vi "Pause.vi"(8 "error in (no error)":errorcluster, 11 "TDCManager":T1) -> (0 "error out":errorcluster, 3 "TDCManager":T1)   [LabVIEW 2016, in "HPTDC Driver Library.lvlib"]
uses:
  HPTDC Driver Library.lvlib
  Typedefs/TDCManager.ctl
  C:/Users/CRT Controller/CRTC Labview Application/Source/HPTDC Driver Library Folder/Library files/hptdc_net4_3.7.0_x64.dll
  hptdc_net4_3.7.0_x64.dll
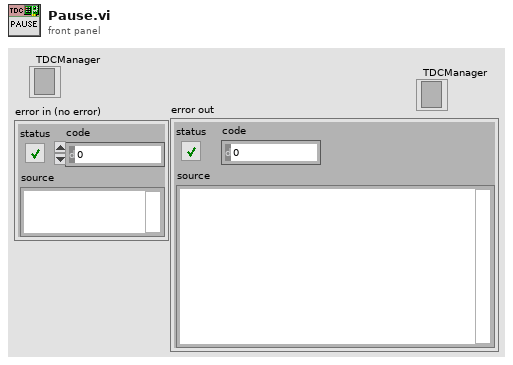
[diagram p1: front panel]
types:
  T1 = typedef "HPTDC Driver Library.lvlib/TDCManager.ctl" = refnum<k24>
  T2 = typedef "Semaphore RefNum" = refnum<k1>
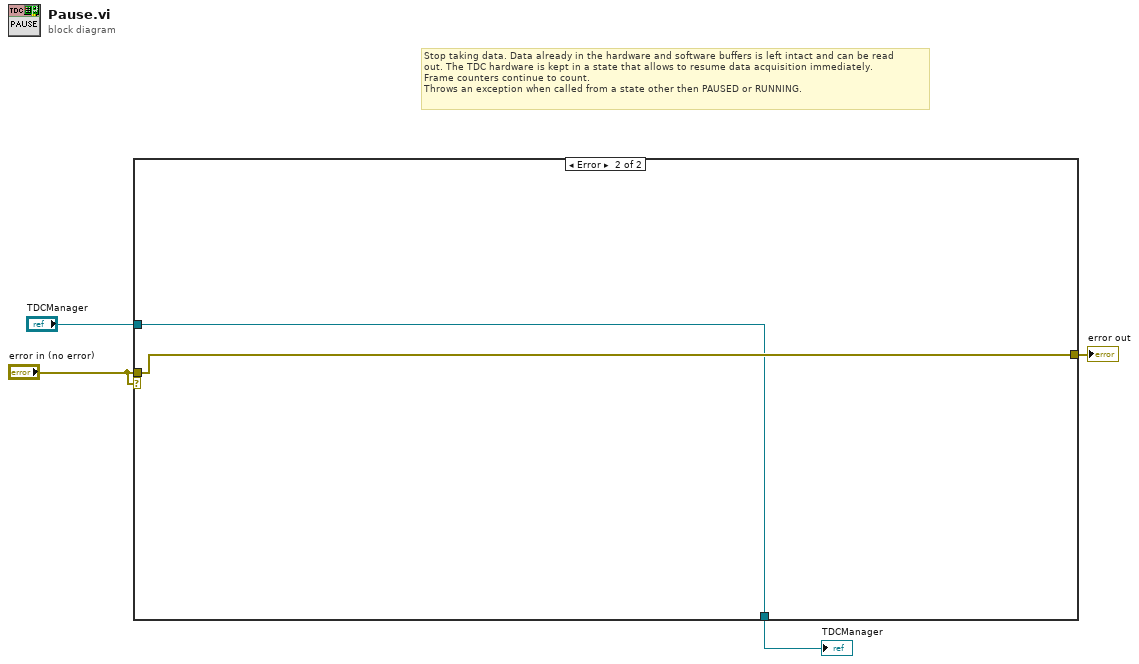
[diagram p0: block diagram]
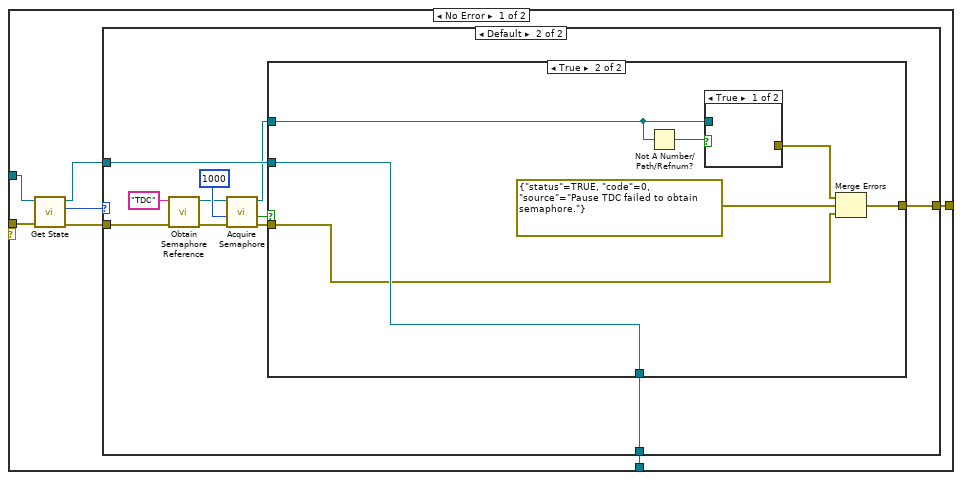
[diagram p2: hidden frame]
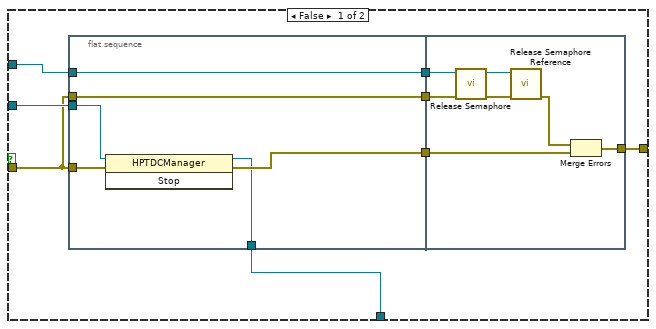
[diagram p4: hidden frame]
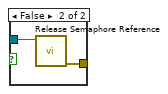
[diagram p5: hidden frame]
diagram:
  # "Stop taking data. Data already in the hardware and software buffers is left intact and can be read\nout. The TDC hardware is kept in a state that allows to resume data acquisition immediately.\nFrame counters continue to count.\nThrows an exception when called from a state other then PAUSED or RUNNING."
  n1 = case shown="Error" "error in (no error)" {
    tunnel: "TDCManager" -> [w11 w55]
    tunnel: "error in (no error)" -> [w10 w56]
    tunnel: [w6 w56] -> w3
    tunnel: [w5 w55] -> w2
    frame No Error {
      n2 = call "Get State.vi"("error in"=w10, "TDCManager"=w11) -> ("error out"=w7:errorcluster, "State"=w9:i32, "TDCManager"=w8:T1)  [unwired: 6 in, 1 out]
      n3 = case shown="Default" w9 {
        tunnel: w7 -> [w13 w19]
        tunnel: w8 -> [w12 w24]
        tunnel: [w12 w15] -> w5
        tunnel: [w13 w14] -> w6
        frame 0..2, 5 {
        }
        frame Default {
          n4 = call <vilib>:"Obtain Semaphore Reference.vi"("error in (no error)"=w19, "name (unnamed)"="TDC") -> ("error out"=w21:errorcluster, "semaphore"=w22:T2)  [unwired: 3 in, 1 out]
          n5 = call <vilib>:"Acquire Semaphore.vi"("error in (no error)"=w21, "ms timeout (-1)"=1000, "semaphore"=w22) -> ("error out"=w17:errorcluster, "timed out"=w18:bool, "semaphore out"=w16:T2)  [unwired: 2 in]
          n6 = case shown="True" w18 {
            tunnel: w24 -> [w32 w52]
            tunnel: w17 -> [w29 w46]
            tunnel: w16 -> [w27 w48]
            tunnel: [w26 w52] -> w15
            tunnel: [w25 w50] -> w14
            frame False {
              n7 = flat-sequence {
                tunnel: w29 -> [w38]
                tunnel: w32 -> [w37]
                tunnel: [w36] -> w31
                tunnel: w29 -> [w35]
                tunnel: [w35] -> w30
                tunnel: [w34] -> w28
                tunnel: w27 -> [w34]
                tunnel: [w33] -> w26
                tunnel: w31 -> [w45]
                tunnel: w30 -> [w42]
                tunnel: w28 -> [w40]
                tunnel: [w39] -> w25
                frame #0 {
                  n8 = invoke class="HPTDCManager" method="Stop"(reference=w37, error in=w38) -> (reference out=w33:T1, error out=w36:errorcluster)  [unwired: 1 in, 1 out]
                }
                frame #1 {
                  n9 = call <vilib>:"Release Semaphore.vi"("error in (no error)"=w42, "semaphore"=w40) -> ("error out"=w43:errorcluster, "semaphore out"=w44:T2)  [unwired: 4 in]
                  n10 = call <vilib>:"Release Semaphore Reference.vi"("error in (no error)"=w43, "semaphore"=w44) -> ("error out"=w41:errorcluster)  [unwired: 8 in, 1 out]
                  n11 = Merge Errors(w41, w45) -> (w39:errorcluster)
                }
              }
            }
            frame True {
              n12 = Not A Number/Path/Refnum?(number/path/refnum=w48) -> (NaN/Path/Refnum?=w47:bool)
              n13 = case shown="True" w47 {
                tunnel: [_ w54] -> w49
                tunnel: w48 -> [_ w53]
                frame True {
                }
                frame False {
                  n14 = call <vilib>:"Release Semaphore Reference.vi"("semaphore"=w53) -> ("error out"=w54:errorcluster)  [unwired: 9 in, 1 out]
                }
              }
              n15 = Merge Errors(w49, errorcluster {"status"=TRUE, "code"=0, "source"="Pause TDC failed to obtain semaphore."} ("error out"), w46) -> (w50:errorcluster)
            }
          }
        }
      }
    }
    frame Error {
    }
  }
  "error out" <- w3
  "TDCManager" <- w2
